vi "Get ASCII.vi"(4 "Source (\"\")":string, 8 "error in (no error)":errorcluster, 11 "VISA resource name":refnum<visa-resource-name>) -> (0 "error out":errorcluster, 2 "ASCII Data":string, 3 "VISA resource name out":refnum<visa-resource-name>)   [LabVIEW 2020, in "Yokogawa GX Series.lvlib"]
doc: "This VI gets ASCII data.\nSend Message, then recieve the response. If Response Type is ASCII, remained datas are recieved by this VI."
uses:
  <instrlib>/Yokogawa GX Series/Yokogawa GX Series.lvlib
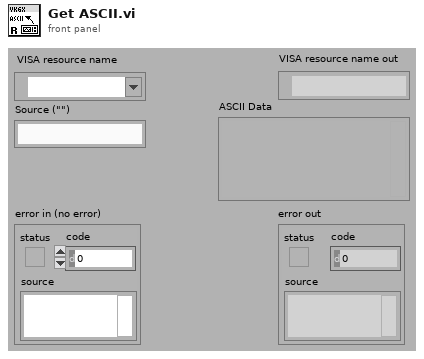
[diagram p1: front panel]
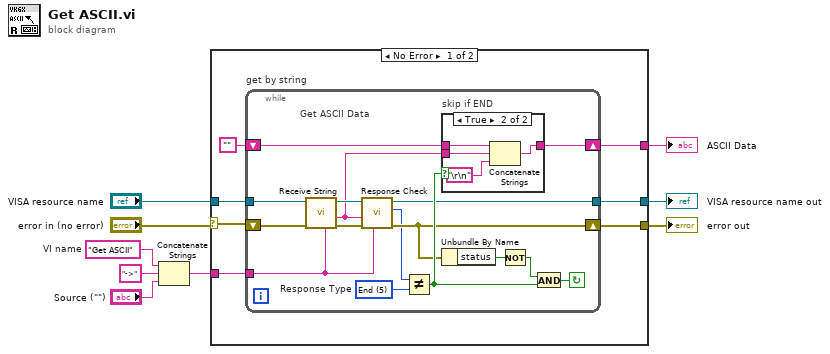
[diagram p0: block diagram]
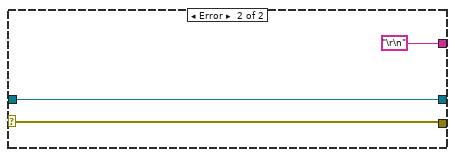
[diagram p3: hidden frame]
diagram:
  w4 = "Get ASCII"  # VI name
  n1 = Concatenate Strings(w4, "->", "Source (\"\")") -> (w5:string)
  n2 = case shown="No Error" "error in (no error)" {
    selector: "error in (no error)" -> [w10 w38]
    tunnel: [w15 w39] -> w9
    tunnel: [w14 "\r\n"] -> w8
    tunnel: "VISA resource name" -> [w13 w39]
    tunnel: [w12 w38] -> w6
    tunnel: w5 -> [w11 _]
    frame No Error {
      n3 = while "get by string" {
        shift-left: w10 -> [w25]
        shift-right: [w20] -> w12
        shift-left: "" -> [w32]
        shift-right: [w31] -> w14
        tunnel: w11 -> [w21]
        tunnel: w13 -> [w26]
        tunnel: [w19] -> w15
        stop <- w29 continue-if-true
        w17 = 5 items=["Affirmative", "Single Negative", "Multiple Negative", "ASCII", "Binary", "End"]  # Response Type
        # "Get ASCII Data"
        n4 = call <instrlib>:"Receive String.vi"("Source (\"\")"=w21, "error in (no error)"=w25, "VISA resource name"=w26) -> ("error out"=w23:errorcluster, "Read Buffer"=w22:string, "VISA resource name out"=w24:refnum<visa-resource-name>)  [unwired: 6 in]
        n5 = call <instrlib>:"Response Check.vi"("Source (\"\")"=w21, "error in (no error)"=w23, "Message In (\"\")"=w22, "VISA resource name"=w24) -> ("error out"=w20:errorcluster, "Response Type"=w18:i32, "VISA resource name out"=w19:refnum<visa-resource-name>)  [unwired: 3 in, 2 out]
        n6 = Not Equal?(x=w18, y=w17) -> (x != y?=w28:bool)
        n7 = case "skip if END" shown="True" w28 {
          tunnel: [w33 w37] -> w31
          tunnel: w32 -> [w33 w36]
          tunnel: w22 -> [_ w35]
          frame False {
          }
          frame True {
            n8 = Concatenate Strings(w36, w35, "\r\n") -> (w37:string)
          }
        }
        n9 = Unbundle By Name(w20) -> ("status"=w30:bool)
        n10 = Not(x=w30) -> (.not. x?=w27:bool)
        n11 = And(x=w27, y=w28) -> (x .and. y?=w29:bool)
      }
    }
    frame Error {
    }
  }
  "error out" <- w6
  "VISA resource name out" <- w9
  "ASCII Data" <- w8
